vi "(SubVI) Remove Zero _YCC.vi"(4 "Array in":dbl[](array[numeric])) -> (1 "Array out":dbl[](array[numeric]))   [LabVIEW 2014]
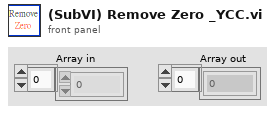
[diagram p1: front panel]
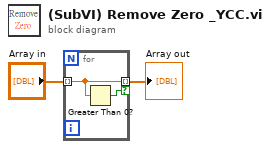
[diagram p0: block diagram]
diagram:
  n1 = for {
    tunnel: "Array in" -> [w3] mode=indexing
    tunnel: [w3] -> w2 mode=indexing if=w4
    n2 = Greater Than 0?(x=w3) -> (x > 0?=w4:bool)
  }
  "Array out" <- w2
